vi "Parse Tokens.vi"(7 "Loader":refnum<class "Abstract.lvclass">, 8 "Error In":errorcluster, 10 "Tokens":refnum<class "Abstract.lvclass">[](array[class]), 11 "Stack In":refnum<queue>) -> (0 "Error Out":errorcluster, 3 "Stack Out":refnum<queue>)   [LabVIEW 2018, in "Toolkit.lvlib"]
uses:
  Toolkit.lvlib
  Nodes/NonTerminal/NonTerminal.lvclass
  Tokens/Abstract/Abstract.lvclass
  Loaders/Abstract/Abstract.lvclass
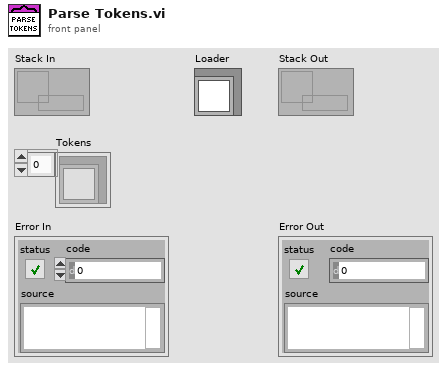
[diagram p1: front panel]
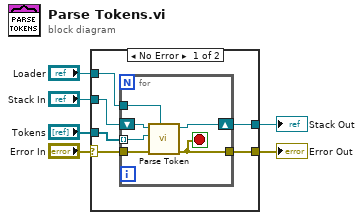
[diagram p0: block diagram]
diagram:
  n1 = case shown="No Error" "Error In" {
    selector: "Error In" -> [w8 w19]
    tunnel: [w12 w20] -> w6
    tunnel: "Stack In" -> [w11 w20]
    tunnel: "Tokens" -> [w10 _]
    tunnel: [w9 w19] -> w3
    tunnel: "Loader" -> [w7 _]
    frame No Error {
      n2 = for {
        tunnel: w10 -> [w14] mode=indexing
        tunnel: w8 -> [w18]
        tunnel: [w17] -> w9
        shift-right: [w16] -> w12
        shift-left: w11 -> [w15]
        tunnel: w7 -> [w13]
        stop <- w17 stop-if-true
        n3 = call "Parse Token.vi"("Loader"=w13, "Error In"=w18, "Token"=w14, "Stack In"=w15) -> ("Error Out"=w17:errorcluster, "Stack Out"=w16:refnum<queue>)  [unwired: 6 in]
      }
    }
    frame Error {
    }
  }
  "Stack Out" <- w6
  "Error Out" <- w3
